vi "Acquire Data.vi"(8 "error in (no error)":errorcluster, 10 "fs notifier":refnum<notifier>, 11 "cam notifier":refnum<notifier>) -> (0 "error out":errorcluster, 1 "force (V)":dbl, 2 "diameter (mm)":dbl, 3 "image":T1, 5 "cam timed out?":bool)   [LabVIEW 2020]
uses:
  Hardware/Sensors/Force Sensors/Force Sensor.lvclass
  <vilib>/vision/Image Controls.llb/IMAQ Image.ctl
  Hardware/Sensors/Cameras/Camera.lvclass
  Hardware/Sensors/Cameras/Camera.lvclass/Camera.ctl
  Hardware/Sensors/Force Sensors/Force Sensor.lvclass/Force Sensor.ctl
  Hardware/Read timestamp.vi
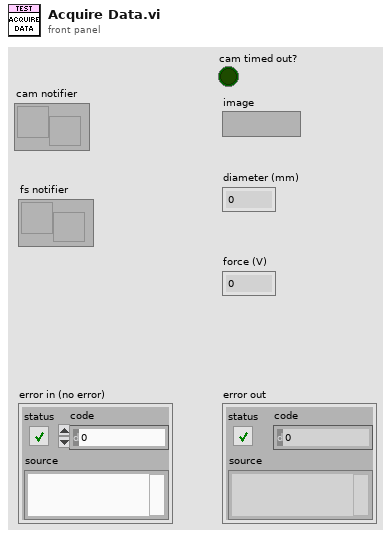
[diagram p1: front panel]
types:
  T1 = typedef "IMAQ Image.ctl" = refnum<image>
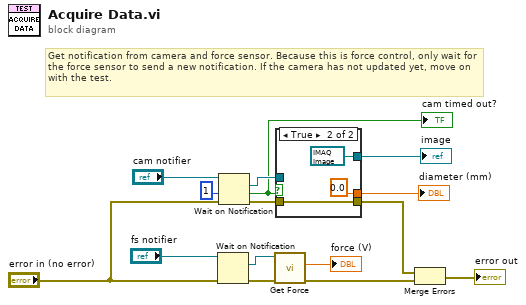
[diagram p0: block diagram]
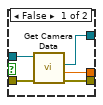
[diagram p2: hidden frame]
diagram:
  # "Get notification from camera and force sensor. Because this is force control, only wait for the force sensor to send a new notification. If the camera has not updated yet, move on with the test."
  n1 = Wait on Notification(notifier="fs notifier", error in (no error)="error in (no error)") -> (notification=w11:refnum<class "Force Sensor.lvclass">, error out=w12:errorcluster)  [unwired: 2 in, 2 out]
  n2 = Wait on Notification(notifier="cam notifier", timeout in ms (-1)=1, error in (no error)="error in (no error)") -> (notification=w7:refnum<class "Camera.lvclass">, timed out?=w4:bool, error out=w8:errorcluster)  [unwired: 1 in, 1 out]
  "cam timed out?" <- w4
  n3 = call "Get Force.vi"("error in (no error)"=w12, "Force Sensor in"=w11) -> ("error out"=w3:errorcluster, "force (V)"=→"force (V)":dbl)  [unwired: 7 in, 1 out]
  n4 = case shown="True" w4 {
    tunnel: [w20 0.0 ("diameter (mm)")] -> w14
    tunnel: [w19 T1 refnum ("image")] -> w9
    tunnel: w8 -> [w18 w21]
    tunnel: w7 -> [w17 _]
    tunnel: [w16 w21] -> w2
    frame False {
      n5 = call "Get Camera Data.vi"("error in (no error)"=w18, "Camera in"=w17) -> ("error out"=w16:errorcluster, "diameter (mm)"=w20:dbl, "image"=w19:T1)  [unwired: 5 in, 2 out]
    }
    frame True {
    }
  }
  "diameter (mm)" <- w14
  "image" <- w9
  n6 = Merge Errors(w2, w3) -> (→"error out":errorcluster)
